vi "Make Writable.vi"   [LabVIEW 2015, in "UniquifyFullyQualifiedVIName.lvclass"]
uses:
  UniquifyFullyQualifiedVIName.lvclass
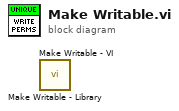
[diagram p0: block diagram]
diagram:
  n1 = call "Make Writable - Library.vi"() -> ()  [unwired: 10 in, 2 out]
  n2 = call "Make Writable - VI.vi"() -> ()  [unwired: 10 in, 2 out]
